vi "API Solen Action.vi"(9 "statue":i32, 11 "solenNum":i32) -> (3 "solenaction return value":bool)   [LabVIEW 2011, in "API DYM.lvlib"]
uses:
  API DYM.lvlib
  DyMechnicalPlatform.dll
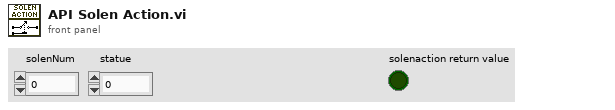
[diagram p1: front panel]
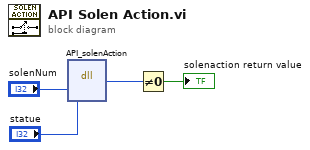
[diagram p0: block diagram]
diagram:
  n1 = dll-call lib="PTH1Xabs D可重构机电平台项目DemoLabViewDYSYSAPIDyMechnicalPlatform.dll" fn="API_solenAction"("solenNum"="solenNum", "statue"="statue") -> ("solenaction return value"=w2:i32)  [unwired: 5 in, 2 out]
  n2 = Not Equal To 0?(x=w2) -> (x != 0?=→"solenaction return value":bool)
